vi "Get Object Refs from Node.vi.vi"(8 "error in":errorcluster, 11 "node ref":T2) -> (0 "error out":errorcluster, 3 "Node object refs":T1)   [LabVIEW 2013, in "Table Manager.lvlib" / "Table Manager.lvclass"]
doc: "This VI gets the Engine reference and cast the node to config node."
uses:
  Table Manager.lvclass
  <vilib>/NI/Configuration Framework/Node/NodeRef.ctl
  <vilib>/NI/Configuration Framework/Node/NISE_CEF_Node.lvclass
  object ref.ctl
  Configuration Editor/Classes/Engine Parent/Engine Parent Editor Node.lvclass
  Configuration Editor/Classes/Module editor node/module editor node.lvclass
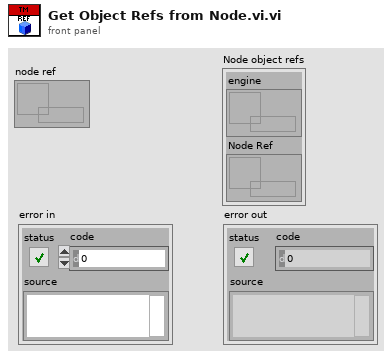
[diagram p1: front panel]
types:
  T1 = typedef "Table Manager.lvlib/Table Manager.lvclass/object ref.ctl" = cluster{"engine":refnum<data-value>, "Node Ref":refnum<data-value>}
  T2 = typedef "NISE_CEF_Node.lvclass/NodeRef.ctl" = refnum<data-value>
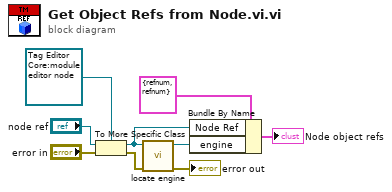
[diagram p0: block diagram]
diagram:
  n1 = To More Specific Class(target class=refnum<data-value> refnum ("data value reference"), reference="node ref", error in="error in") -> (specific class reference=w5:refnum<data-value>, error out=w3:errorcluster)
  n2 = call "locate engine.vi"("error in"=w3, "component"=w5) -> ("error out"=→"error out":errorcluster, "engine"=w6:refnum<data-value>)  [unwired: 8 in]
  n3 = Bundle By Name(cluster=T1 {"engine"=refnum, "Node Ref"=refnum} ("Node object refs"), "Node Ref"=w5, "engine"=w6) -> (→"Node object refs":T1)
